vi "Calibrator.vi"() -> ()   [LabVIEW 2022 SP3]
uses:
  <vilib>/MakerHub/LINX/LMH-LINX.lvlib
  <vilib>/MakerHub/LINX/Public/Peripherals/Analog/Analog Read 1 Chan.vi
  <vilib>/MakerHub/LINX/Public/Peripherals/Analog/Analog Write 1 Chan.vi
panel:
  out "Numeric 2":dbl
  out "Numeric":dbl
  in  "Boolean 2":bool
  out "Boolean":bool
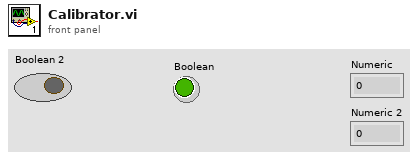
[diagram p1: front panel]
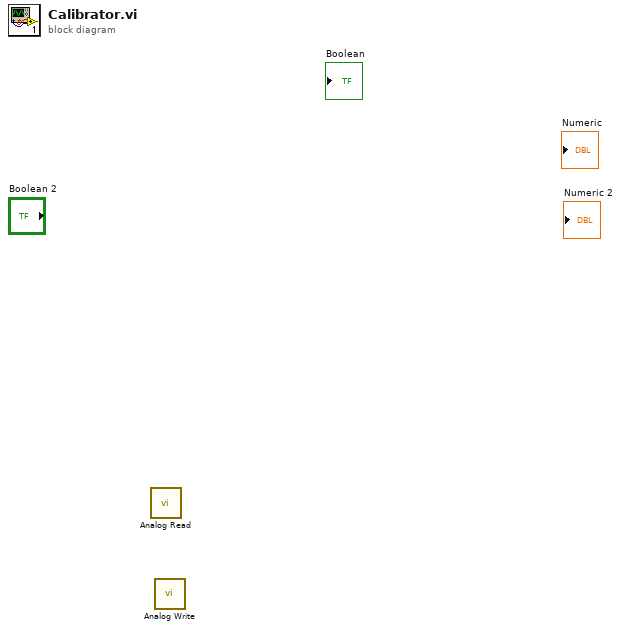
[diagram p0: block diagram]
diagram:
  n1 = call-poly <vilib>:"Analog Read.vi"() -> ()  [unwired: 8 in, 4 out]
  n2 = call-poly <vilib>:"Analog Write.vi"() -> ()  [unwired: 10 in, 2 out]
